vi "hasRam.vi"(0 "Camera in":refnum<class "Camera.lvclass">, 11 "error in (no error)":errorcluster) -> (4 "Camera out":refnum<class "Camera.lvclass">, 6 "hasRam":bool, 15 "error out":errorcluster)   [LabVIEW 2019, in "Camera.lvclass"]
doc: "Determines if the camera has internal memory (camera RAM)"
uses:
  Camera.lvclass
  Camera.lvclass/Camera.ctl
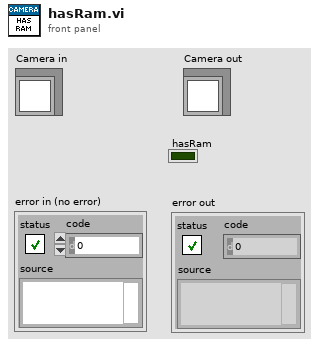
[diagram p1: front panel]
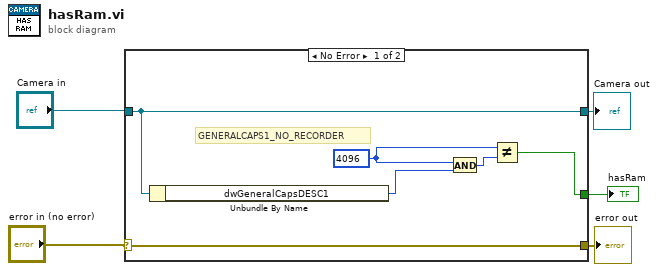
[diagram p0: block diagram]
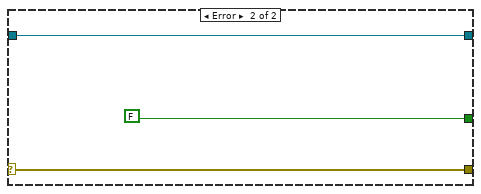
[diagram p2: hidden frame]
diagram:
  n1 = case shown="No Error" "error in (no error)" {
    selector: "error in (no error)" -> [w10 w14]
    tunnel: [w10 w14] -> w3
    tunnel: [w11 w13] -> w4
    tunnel: "Camera in" -> [w11 w13]
    tunnel: [w6 FALSE] -> w1
    frame No Error {
      w7 = u32 4096
      # "GENERALCAPS1_NO_RECORDER"
      n2 = Unbundle By Name(w11) -> ("dwGeneralCapsDESC1"=w9:u32)
      n3 = And(x=w7, y=w9) -> (x .and. y?=w8:u32)
      n4 = Not Equal?(x=w7, y=w8) -> (x != y?=w6:bool)
    }
    frame Error {
    }
  }
  "error out" <- w3
  "Camera out" <- w4
  "hasRam" <- w1
